vi "GetCurrents.vi"(8 "error in (no error)":errorcluster, 10 "Samples":dbl=1024.0, 11 "TecellaChannel in":refnum<class "TecellaChannel.lvclass">) -> (0 "error out":errorcluster, 2 "Currents (nA)":dbl[][](array[numeric]), 3 "TecellaChannel out":refnum<class "TecellaChannel.lvclass">)   [LabVIEW 2009, in "TecellaChannel.lvclass"]
uses:
  TecellaChannel.lvclass
  TecellaChannel.lvclass/TecellaChannel.ctl
  TecellaClient/TecellaClient.lvclass
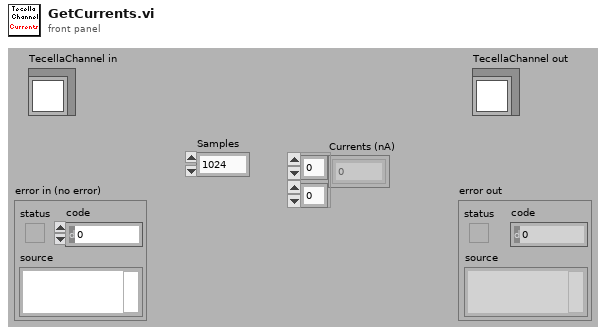
[diagram p1: front panel]
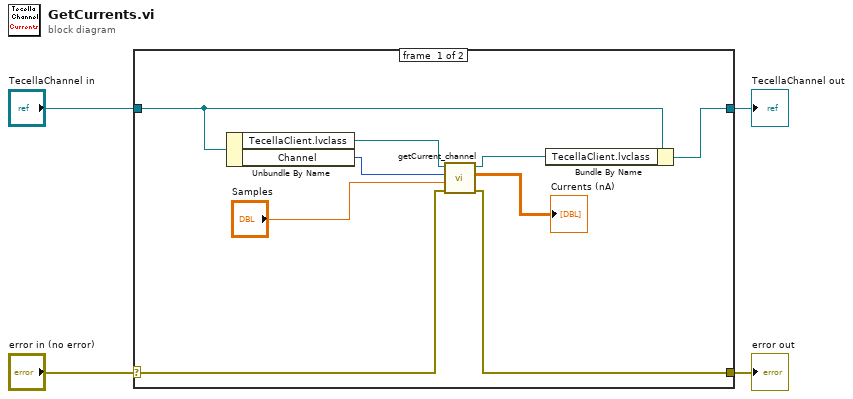
[diagram p0: block diagram]
diagram:
  n1 = case shown="No Error" "error in (no error)" {
    selector: "error in (no error)" -> [w6 w15]
    tunnel: [w5 w15] -> w3
    tunnel: [w12 w14] -> w1
    tunnel: "TecellaChannel in" -> [w13 w14]
    frame #0 {
      n2 = Unbundle By Name(w13) -> ("TecellaClient.lvclass"=w11:refnum<class "TecellaClient.lvclass">, "Channel"=w9:i8)
      n3 = call-dynamic "getCurrent_channel.vi"("error in (no error)"=w6, "Samples"="Samples", "Channel"=w9, "TecellaClient in"=w11) -> ("error out"=w5:errorcluster, "Currents"=→"Currents (nA)":dbl[][], "TecellaClient out"=w10:refnum<class "TecellaClient.lvclass">)  [unwired: 5 in]
      n4 = Bundle By Name(cluster=w13, "TecellaClient.lvclass"=w10) -> (w12:refnum<class "TecellaChannel.lvclass">)
    }
    frame #1 {
    }
  }
  "error out" <- w3
  "TecellaChannel out" <- w1
